vi "Read TCP Ref.vi"(8 "error in (no error)":errorcluster, 11 "Ethernet in":refnum<class "TCP.lvclass">) -> (0 "error out":errorcluster, 2 "TCP Ref":refnum<k5>, 3 "Ethernet out":refnum<class "TCP.lvclass">)   [LabVIEW 2019, in "Protocols.lvlib" / "TCP.lvclass"]
uses:
  TCP.lvclass
  TCP.lvclass/TCP.ctl
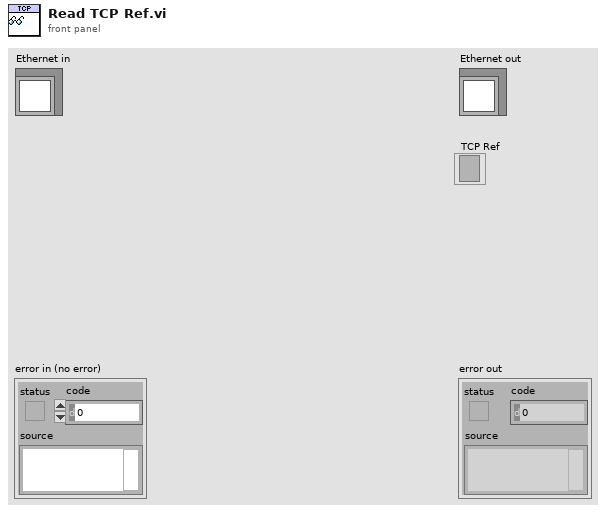
[diagram p1: front panel]
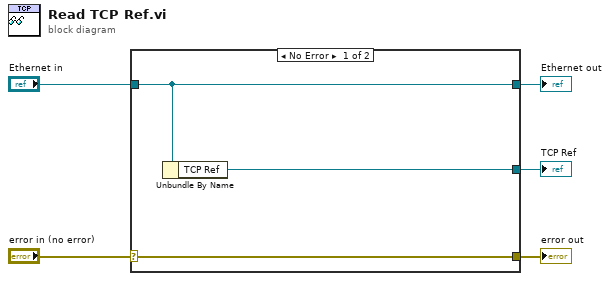
[diagram p0: block diagram]
diagram:
  n1 = case shown="No Error" "error in (no error)" {
    selector: "error in (no error)" -> [w8 w9]
    tunnel: [w8 w9] -> w4
    tunnel: [w7 w10] -> w2
    tunnel: "Ethernet in" -> [w7 w10]
    tunnel: [w6 _] -> w1
    frame No Error {
      n2 = Unbundle By Name(w7) -> ("TCP Ref"=w6:refnum<k5>)
    }
    frame Error {
    }
  }
  "error out" <- w4
  "Ethernet out" <- w2
  "TCP Ref" <- w1
